vi "AMI_Compara_Min_Indices.vi"() -> (1 "Min_idx":i16, 6 "idxScanVi":i16, 8 "idxScanTi":i16, 9 "idxScanXi":i16, 10 "idxScanYi":i16, 11 "idxScanZi":i16)   [LabVIEW 2017]
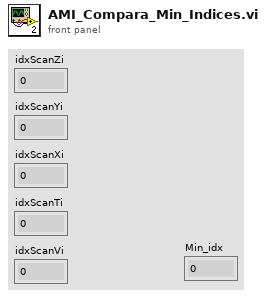
[diagram p1: front panel]
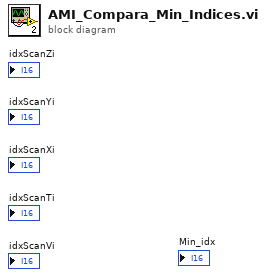
[diagram p0: block diagram]
diagram:
